vi "4led_driver.vi"(1 "4led signal":dbl) -> (0 "colorbox":u32)   [LabVIEW 2017]
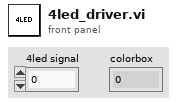
[diagram p1: front panel]
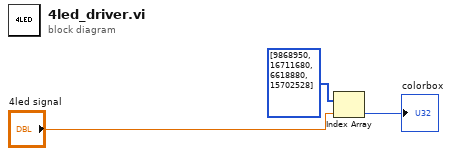
[diagram p0: block diagram]
diagram:
  n1 = Index Array(array=u32[] [9868950, 16711680, 6618880, 15702528], index="4led signal") -> (element=→"colorbox":u32)
